vi "PH_StatusHandler.set i Attr and create DIM services.vi"(0 "VI in":refnum<vi>, 5 "error in (no error)":errorcluster) -> (14 "VI out":refnum<vi>, 16 "i attribute":T1 {"Value" items=["no info", "off/false/out", "on/true/in", "Failure", "Alarm", "Status 1", "Status 2", "Status 3"]}, 19 "error out":errorcluster)   [LabVIEW 2014, in "PH_StatusHandler.lvlib"]
uses:
  PH_StatusHandler.lvlib
  PH_StatusHandler.i attribute.ctl
  PH_StatusHandler.GUI element.ctl
  PH_StatusHandler.Status.ctl
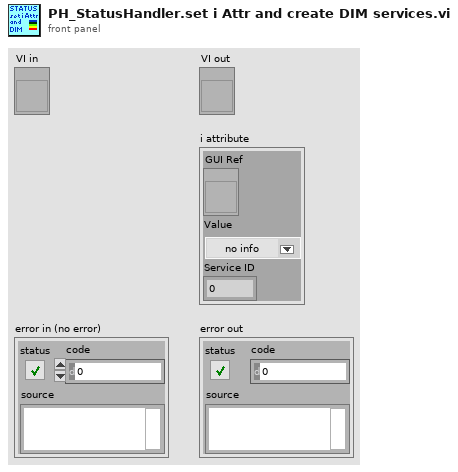
[diagram p1: front panel]
types:
  T1 = typedef "PH_StatusHandler.lvlib/PH_StatusHandler.i attribute.ctl" = cluster{"GUI Ref":refnum<vi>, "Value":T2, "Service ID":i32}
  T2 = typedef "PH_StatusHandler.lvlib/PH_StatusHandler.Status.ctl" = i16
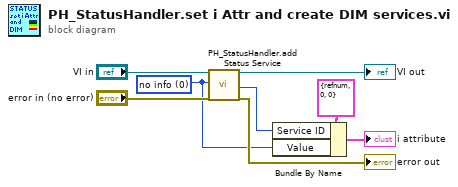
[diagram p0: block diagram]
diagram:
  w1 = T2 0 items=["no info", "off/false/out", "on/true/in", "Failure", "Alarm", "Status 1", "Status 2", "Status 3"] ("Status")
  n1 = call "PH_StatusHandler.add Status Service.vi"("i ref in"="VI in", "Status"=w1, "error in (no error)"="error in (no error)") -> ("i ref out"=→"VI out":refnum<vi>, "Service ID Status"=w2:i32, "error out"=→"error out":errorcluster)  [unwired: 14 in]
  n2 = Bundle By Name(cluster=T1 {"GUI Ref"=refnum, "Value"=0, "Service ID"=0} ("i attribute"), "Service ID"=w2, "Value"=w1) -> (→"i attribute":T1)
